vi "programacion paralela.vi"() -> ()   [LabVIEW 2020]
panel:
  out "Tank 8":u8(slide) scale=0.0..100.0
  out "Tank 7":u8(slide) scale=0.0..100.0
  out "Tank 6":u8(slide) scale=0.0..100.0
  out "Tank 5":u8(slide) scale=0.0..100.0
  out "Tank 4":u8(slide) scale=0.0..100.0
  out "Tank 3":u8(slide) scale=0.0..100.0
  out "Tank 2":u8(slide) scale=0.0..100.0
  out "Tank 1":u8(slide) scale=0.0..100.0
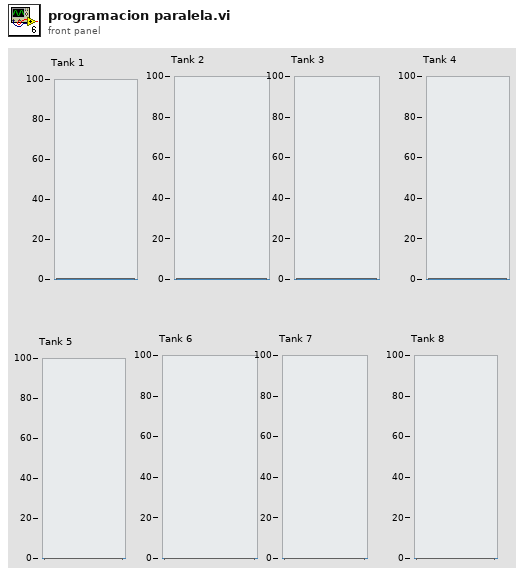
[diagram p1: front panel]
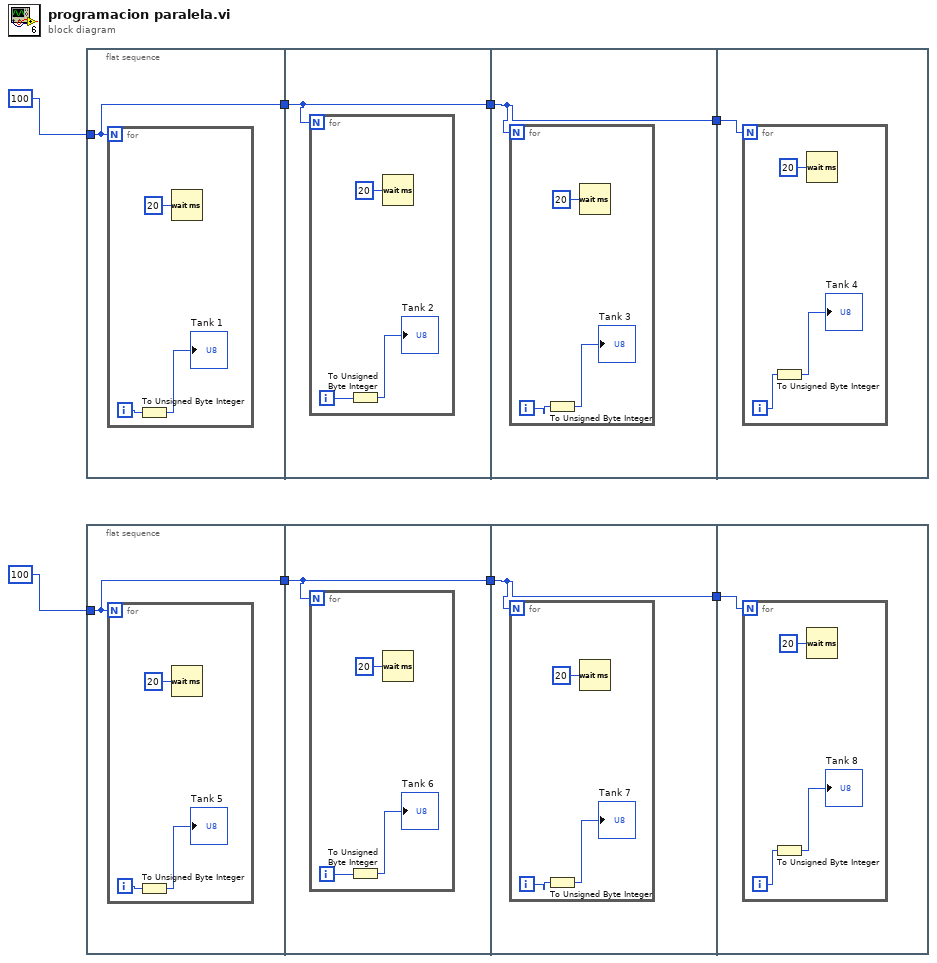
[diagram p0: block diagram]
diagram:
  n1 = flat-sequence {
    tunnel: 100 -> [w9]
    tunnel: [w9] -> w8
    tunnel: w8 -> [w13]
    tunnel: [w13] -> w7
    tunnel: w7 -> [w17]
    tunnel: [w17] -> w6
    tunnel: w6 -> [w21]
    frame #0 {
      n2 = for {
        N: w9 -> [_]
        i -> [w12]
        n3 = To Unsigned Byte Integer(number=w12) -> (unsigned 8bit integer=→"Tank 1":u8)
        n4 = Wait (ms)(milliseconds to wait=u32 20) -> ()  [unwired: 1 out]
      }
    }
    frame #1 {
      n5 = for {
        N: w13 -> [_]
        i -> [w14]
        n6 = To Unsigned Byte Integer(number=w14) -> (unsigned 8bit integer=→"Tank 2":u8)
        n7 = Wait (ms)(milliseconds to wait=u32 20) -> ()  [unwired: 1 out]
      }
    }
    frame #2 {
      n8 = for {
        N: w17 -> [_]
        i -> [w18]
        n9 = To Unsigned Byte Integer(number=w18) -> (unsigned 8bit integer=→"Tank 3":u8)
        n10 = Wait (ms)(milliseconds to wait=u32 20) -> ()  [unwired: 1 out]
      }
    }
    frame #3 {
      n11 = for {
        N: w21 -> [_]
        i -> [w22]
        n12 = To Unsigned Byte Integer(number=w22) -> (unsigned 8bit integer=→"Tank 4":u8)
        n13 = Wait (ms)(milliseconds to wait=u32 20) -> ()  [unwired: 1 out]
      }
    }
  }
  n14 = flat-sequence {
    tunnel: 100 -> [w25]
    tunnel: [w25] -> w4
    tunnel: w4 -> [w29]
    tunnel: [w29] -> w3
    tunnel: w3 -> [w33]
    tunnel: [w33] -> w2
    tunnel: w2 -> [w37]
    frame #0 {
      n15 = for {
        N: w25 -> [_]
        i -> [w28]
        n16 = To Unsigned Byte Integer(number=w28) -> (unsigned 8bit integer=→"Tank 5":u8)
        n17 = Wait (ms)(milliseconds to wait=u32 20) -> ()  [unwired: 1 out]
      }
    }
    frame #1 {
      n18 = for {
        N: w29 -> [_]
        i -> [w30]
        n19 = To Unsigned Byte Integer(number=w30) -> (unsigned 8bit integer=→"Tank 6":u8)
        n20 = Wait (ms)(milliseconds to wait=u32 20) -> ()  [unwired: 1 out]
      }
    }
    frame #2 {
      n21 = for {
        N: w33 -> [_]
        i -> [w34]
        n22 = To Unsigned Byte Integer(number=w34) -> (unsigned 8bit integer=→"Tank 7":u8)
        n23 = Wait (ms)(milliseconds to wait=u32 20) -> ()  [unwired: 1 out]
      }
    }
    frame #3 {
      n24 = for {
        N: w37 -> [_]
        i -> [w38]
        n25 = To Unsigned Byte Integer(number=w38) -> (unsigned 8bit integer=→"Tank 8":u8)
        n26 = Wait (ms)(milliseconds to wait=u32 20) -> ()  [unwired: 1 out]
      }
    }
  }
